vi "Configure.vi"(8 "error in":errorcluster, 10 "Output Settings":T1={"Voltage (V)"=1.0} {"Voltage (V)" min=-424.2 max=424.2 step=1.0 format="%#.1f"}, 11 "VISA Interface in":refnum<class "VISA Interface.lvclass">) -> (0 "error out":errorcluster, 3 "VISA Interface out":refnum<class "VISA Interface.lvclass">)   [LabVIEW 2020, in "Plugin Instrument Driver.lvlib" / "VISA Interface.lvclass"]
doc: "Set Output channel"
uses:
  VISA Interface.lvclass
  Typedefs/Output Settings.ctl
  Instrument Driver.lvclass
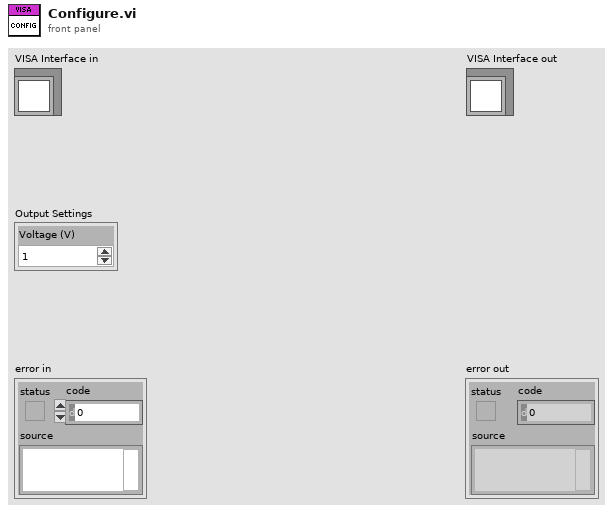
[diagram p1: front panel]
types:
  T1 = typedef "Plugin Instrument Driver.lvlib/Instrument Driver.lvclass/Output Settings.ctl" = cluster{"Voltage (V)":dbl}
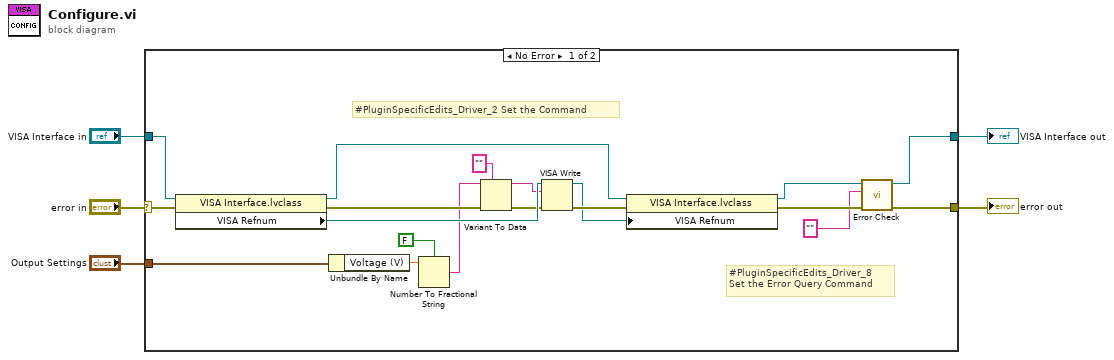
[diagram p0: block diagram]
diagram:
  n1 = case shown="No Error" "error in" {
    selector: "error in" -> [w23 w25]
    tunnel: "VISA Interface in" -> [w24 w26]
    tunnel: [w8 w25] -> w3
    tunnel: [w10 w26] -> w2
    tunnel: "Output Settings" -> [w12 _]
    frame No Error {
      # "#PluginSpecificEdits_Driver_8\nSet the Error Query Command"
      # "#PluginSpecificEdits_Driver_2 Set the Command"
      n2 = property class="VISA Interface.lvclass"(reference=w24, error in=w23) -> (reference out=w21:refnum<class "VISA Interface.lvclass">, error out=w18:errorcluster, "VISA Refnum"=w22:refnum<visa-resource-name>)
      n3 = Unbundle By Name(w12) -> ("Voltage (V)"=w14:dbl)
      n4 = Number To Fractional String(use system decimal point (T)=FALSE, number=w14) -> (F-format string=w13:string)  [unwired: 2 in]
      n5 = Variant To Data(error in=w18, type="" ("write buffer"), Variant=w13) -> (data=w15:string, error out=w17:errorcluster)
      n6 = VISA Write(VISA resource name=w22, write buffer=w15, error in (no error)=w17) -> (VISA resource name out=w19:refnum<visa-resource-name>, error out=w20:errorcluster)  [unwired: 1 out]
      n7 = property class="VISA Interface.lvclass"(reference=w21, error in=w20, "VISA Refnum"=w19) -> (reference out=w11:refnum<class "VISA Interface.lvclass">, error out=w9:errorcluster)
      n8 = call "Error Check.vi"("error in"=w9, "Error Query Command"="", "VISA Interface in"=w11) -> ("error out"=w8:errorcluster, "VISA Interface out"=w10:refnum<class "VISA Interface.lvclass">)  [unwired: 7 in]
    }
    frame Error {
    }
  }
  "error out" <- w3
  "VISA Interface out" <- w2
